vi "FRCts20_Backend_API_EventRoot.vi"(8 "error in (no error)":errorcluster, 10 "Message":T2="GetEventRoot", 11 "EventRoot In":T1) -> (0 "error out":errorcluster, 2 "Status":string, 3 "EventRoot Out":T1)   [LabVIEW 2013, in "FRCts20_Backend_API.lvlib"]
doc: "This API call either returns data for all events (including the number of open issues and which are live) or creates a new event"
uses:
  FRCts20_Backend_API.lvlib
  FRCts20_Backend_API_EventRoot.ctl
  FRCts20_Backend_API_Command_EventRoot.ctl
  FRCts20_Backend_FGVOperation.ctl
  FRCts20_Backend_Engine.lvlib
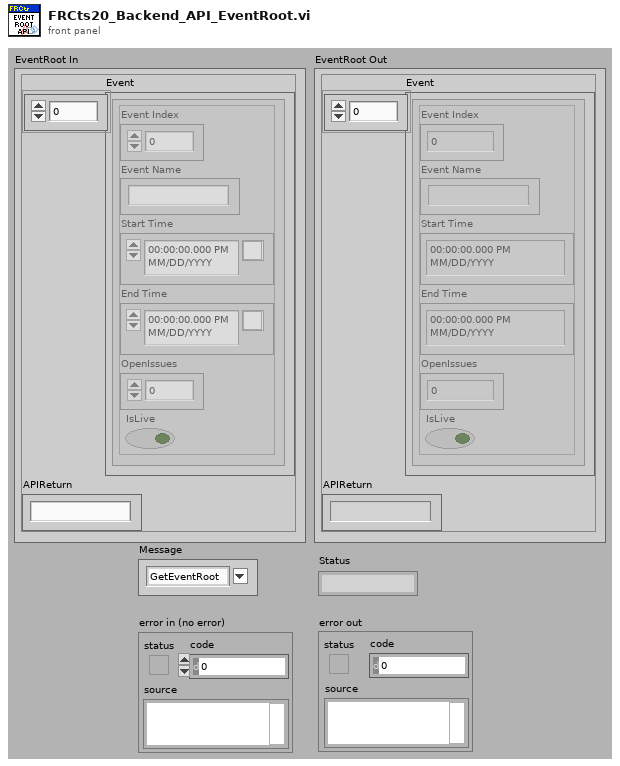
[diagram p1: front panel]
types:
  T1 = typedef "FRCts20_Backend_API.lvlib/FRCts20_Backend_API_EventRoot.ctl" = cluster{"Event":cluster{"Event Index":u32, "Event Name":string, "Start Time":timestamp, "End Time":timestamp, "OpenIssues":u8, "IsLive":bool}[], "APIReturn":string}
  T2 = typedef "FRCts20_Backend_API.lvlib/FRCts20_Backend_API_Command_EventRoot.ctl" = string
  T3 = typedef "FRCts20_Backend_Engine.lvlib/FRCts20_Backend_FGVOperation.ctl" = enum16{"Initialize", "EnqueueMessage", "EnqueueDataReturn", "FlushMessage", "FlushDataReturn"}
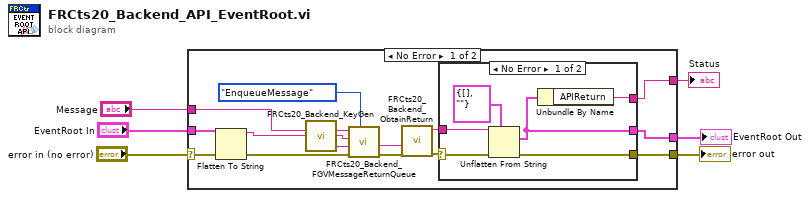
[diagram p0: block diagram]
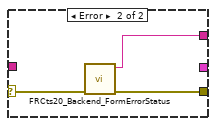
[diagram p2: hidden frame]
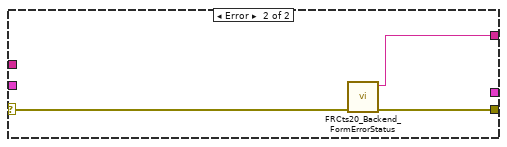
[diagram p3: hidden frame]
diagram:
  n1 = case shown="No Error" "error in (no error)" {
    selector: "error in (no error)" -> [w10 w32]
    tunnel: [w12 w31] -> w5
    tunnel: [w14 w30] -> w4
    tunnel: [w13 _] -> w3
    tunnel: "Message" -> [w16 _]
    tunnel: "EventRoot In" -> [w9 _]
    frame No Error {
      n2 = Flatten To String(anything=w9, error in (no error)=w10) -> (data string=w8:string, error out=w7:errorcluster)  [unwired: 2 in, 1 out]
      n3 = call "FRCts20_Backend_KeyGen.vi"() -> ("Keygen"=w20:string)  [unwired: 27 in]
      n4 = call "FRCts20_Backend_FGVMessageReturnQueue.vi"("Operation"=FRCts20_Backend_FGVOperation."EnqueueMessage", "error in (no error)"=w7, "Key"=w20, "Message Value"=w8, "Message Name"=w16) -> ("error out"=w18:errorcluster, "Key (Duplicate)"=w17:string)  [unwired: 5 in]
      n5 = call "FRCts20_Backend_ObtainReturn.vi"("error in (no error)"=w18, "Key"=w17) -> ("error out"=w15:errorcluster, "Message Value"=w11:string)  [unwired: 8 in]
      n6 = case shown="No Error" w15 {
        selector: w15 -> [w25 w27]
        tunnel: [w26 w28] -> w12
        tunnel: [w24 _] -> w13
        tunnel: [w23 w29] -> w14
        tunnel: w11 -> [w21 _]
        frame No Error {
          n7 = Unflatten From String(type=T1 {"Event"=[], "APIReturn"=""} ("Competitions"), binary string=w21, error in (no error)=w25) -> (value=w24:T1, error out=w26:errorcluster)  [unwired: 2 in, 1 out]
          n8 = Unbundle By Name(w24) -> ("APIReturn"=w23:string)
        }
        frame Error {
          n9 = call "FRCts20_Backend_FormErrorStatus.vi"("error in (no error)"=w27) -> ("error out"=w28:errorcluster, "String"=w29:string)  [unwired: 9 in]
        }
      }
    }
    frame Error {
      n10 = call "FRCts20_Backend_FormErrorStatus.vi"("error in (no error)"=w32) -> ("error out"=w31:errorcluster, "String"=w30:string)  [unwired: 9 in]
    }
  }
  "error out" <- w5
  "Status" <- w4
  "EventRoot Out" <- w3
